vi "Save Image as TIFF.vi"(7 "prompt":string, 8 "error in (no error)":errorcluster, 9 "Default Name":string, 10 "File Path in (Empty: Dialog)":path, 11 "Image Refnum in":T1) -> (0 "error out":errorcluster, 1 "Message":string, 2 "File Path out":path, 4 "Cancelled?":bool)   [LabVIEW 2021, in "Image.lvlib"]
uses:
  <vilib>/vision/Image Controls.llb/IMAQ Image.ctl
  Image.lvlib
  Files/Files.lvlib
  Strings/Strings.lvlib
panel:
  out "Image Out (dup)":T1
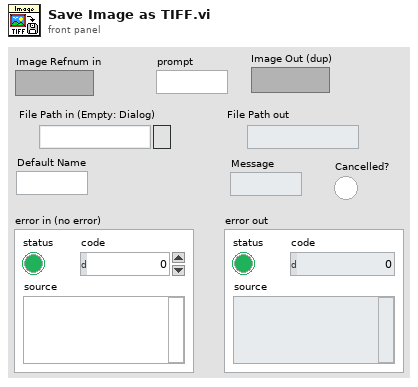
[diagram p1: front panel]
types:
  T1 = typedef "IMAQ Image.ctl" = refnum<image>
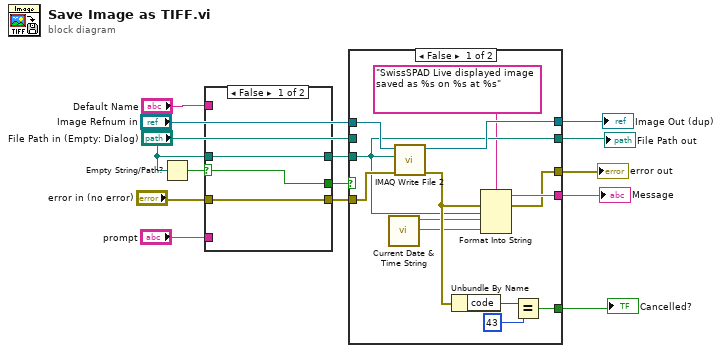
[diagram p0: block diagram]
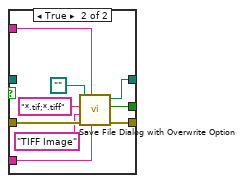
[diagram p3: hidden frame]
diagram:
  n1 = Empty String/Path?(string/path="File Path in (Empty: Dialog)") -> (empty?=w10:bool)
  n2 = case shown="False" w10 {
    selector: w10 -> [w16 _]
    tunnel: "error in (no error)" -> [w15 w26]
    tunnel: [w15 w25] -> w8
    tunnel: [w16 w24] -> w7
    tunnel: "File Path in (Empty: Dialog)" -> [w17 _]
    tunnel: [w17 w23] -> w4
    tunnel: "Default Name" -> [_ w22]
    tunnel: "prompt" -> [_ w19]
    frame False {
    }
    frame True {
      n3 = call "Save File Dialog with Overwrite Option.vi"("prompt"=w19, "Default Name"=w22, "error in (no error)"=w26, "pattern label"="TIFF Image", "pattern (all files)"="*.tif;*.tiff", "Starting Folder"=path "") -> ("error out"=w25:errorcluster, "cancelled"=w24:bool, "selected path"=w23:path)  [unwired: 2 in, 1 out]
    }
  }
  n4 = case shown="False" w7 {
    selector: w7 -> [_ w43]
    tunnel: "Image Refnum in" -> [w39 w41]
    tunnel: [w38 w41] -> w13
    tunnel: [w31 w42] -> w12
    tunnel: [w35 w43] -> w11
    tunnel: w8 -> [w34 w42]
    tunnel: "File Path in (Empty: Dialog)" -> [_ w40]
    tunnel: [w30 w40] -> w6
    tunnel: w4 -> [w30 _]
    tunnel: [w33 _] -> w1
    frame False {
      n5 = call "Current Date & Time String.vi"() -> ("time string"=w27:string, "date string"=w28:string)  [unwired: 9 in, 1 out]
      n6 = call-poly "IMAQ Write File 2"("error in (no error)"=w34, "File Path"=w30, "Image"=w39) -> ("error out"=w32:errorcluster, "Image Out (duplicate)"=w38:T1)  [unwired: 7 in]
      n7 = Unbundle By Name(w32) -> ("code"=w37:i32)
      n8 = Format Into String(format string="SwissSPAD Live displayed image saved as %s on %s at %s", error in=w32, w30, w28, w27) -> (resulting string=w33:string, error out=w31:errorcluster)  [unwired: 1 in]
      n9 = Equal?(x=w37, y=43) -> (x = y?=w35:bool)
    }
    frame True {
    }
  }
  "Message" <- w1
  "error out" <- w12
  "File Path out" <- w6
  "Cancelled?" <- w11
  "Image Out (dup)" <- w13
